vi "CleanUp.vi"(8 "error in (no error)":errorcluster, 11 "imuSensor in":refnum<class "imuSensor.lvclass">) -> (0 "error out":errorcluster, 3 "imuSensor out":refnum<class "imuSensor.lvclass">)   [LabVIEW 2020, in "RPI.SenseHat.Sensors.lvlib" / "imuSensor.lvclass"]
uses:
  imuSensor.lvclass
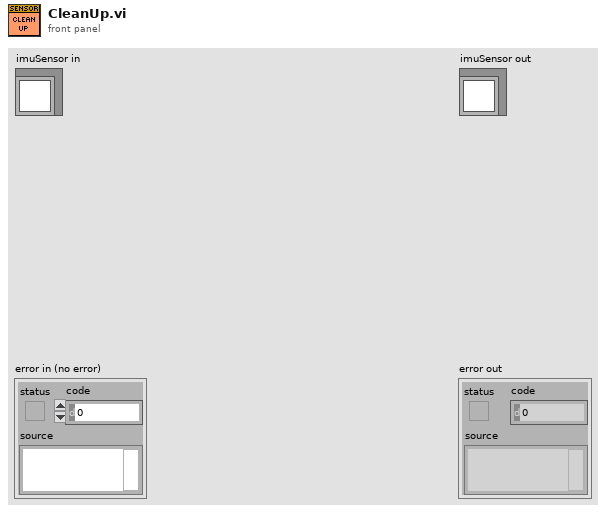
[diagram p1: front panel]
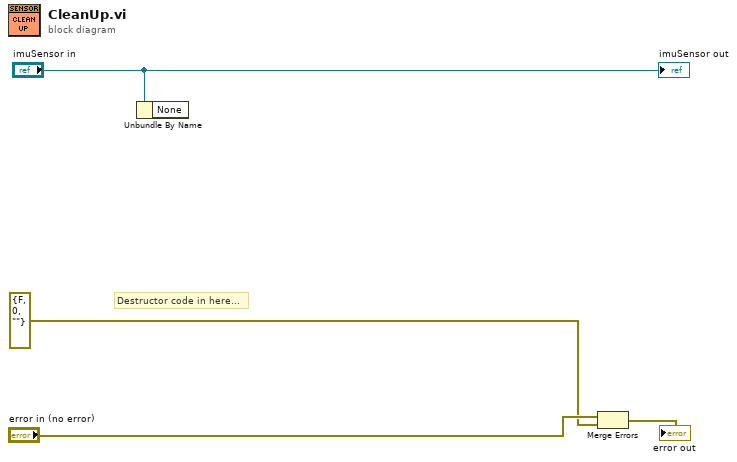
[diagram p0: block diagram]
diagram:
  # "Destructor code in here..."
  n1 = Unbundle By Name("imuSensor in") -> ()  [unwired: 1 out]
  n2 = Merge Errors("error in (no error)", errorcluster {"status"=FALSE, "code"=0, "source"=""} ("error in (no error)")) -> (→"error out":errorcluster)
  "imuSensor out" <- "imuSensor in"
